vi "Flock_Shared_Read Value.vi"(7 "Stand Alone?":bool, 8 "error in (no error)":errorcluster, 10 "timeout (1ms)":i32=1, 11 "Process":T1) -> (0 "error out":errorcluster, 1 "Message Value":string, 2 "Message Name":string, 3 "Process":T1, 5 "Exit Process":bool)   [LabVIEW 2013, in "Flock_Shared_Messaging.lvlib" / "Flock_Shared_LocalProcessMessaging.lvlib"]
uses:
  Flock_Shared_LocalProcessMessaging.lvlib
  FGV_Action.ctl
  Flock_Shared_Messaging.lvlib
  ProcessList.ctl
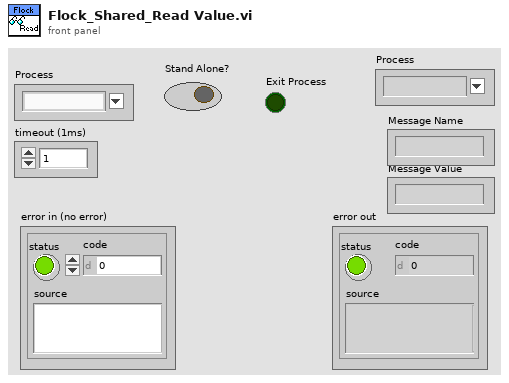
[diagram p1: front panel]
types:
  T1 = typedef "Flock_Shared_Messaging.lvlib/ProcessList.ctl" = string
  T2 = typedef "FGV_Action.ctl" = enum16{"Initalize Central", "Initialize Local", "Get", "Delete Local"}
  T3 = typedef "amc_Message Queue.ctl" = refnum<queue>
  T4 = typedef "Flock_Shared_Messaging.lvlib/FGV_Queues.ctl" = cluster{"Local Queue in 2":T3, "Enum":T1}[]
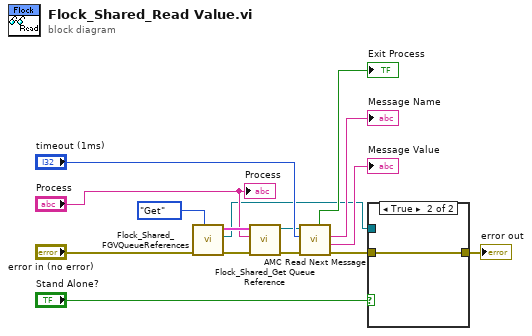
[diagram p0: block diagram]
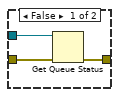
[diagram p2: hidden frame]
diagram:
  n1 = call "Flock_Shared_FGVQueueReferences.vi"("Action"=FGV_Action."Get", "error in (no error)"="error in (no error)") -> ("error out"=w3:errorcluster, "Central Queue out"=w7:T3, "Array"=w12:T4)  [unwired: 7 in]
  n2 = call "Flock_Shared_Get Queue Reference.vi"("Error In"=w3, "Enum"="Process", "Array"=w12) -> ("Error Out"=w5:errorcluster, "Local Queue out"=w6:T3)  [unwired: 7 in]
  n3 = call <vilib>:"AMC Read Next Message.vi"("error in (no error)"=w5, "timeout (1ms)"="timeout (1ms)", "Message Queue in"=w6) -> ("error out"=w2:errorcluster, "Message Value"=→"Message Value":string, "Message Name"=→"Message Name":string, "Exit Process"=→"Exit Process":bool)  [unwired: 2 in, 3 out]
  n4 = case shown="True" "Stand Alone?" {
    tunnel: w7 -> [w18 _]
    tunnel: w2 -> [w17 w19]
    tunnel: [w16 w19] -> w1
    frame False {
      n5 = Get Queue Status(queue=w18, error in (no error)=w17) -> (error out=w16:errorcluster)  [unwired: 1 in, 7 out]
    }
    frame True {
    }
  }
  "error out" <- w1
  "Process" <- "Process"
